vi "head.vi"(8 "error in (no error)":errorcluster, 11 "KNR in":T1) -> (0 "error out":errorcluster, 3 "KNR out":T1)   [LabVIEW 2013]
uses:
  <userlib>/KNR OS 3.0 LabVIEW Toolkit/Type Definition/KNR3 Reference.ctl
  <userlib>/_FPGA Interface Advanced Tools/FPGA Interface Base/FPGA Interface Base.lvclass
  <userlib>/KNR OS 3.0 LabVIEW Toolkit/Type Definition/Resource.ctl
  <userlib>/KNR OS 3.0 LabVIEW Toolkit/Type Definition/DC Motor Port.ctl
  Global 1.vi
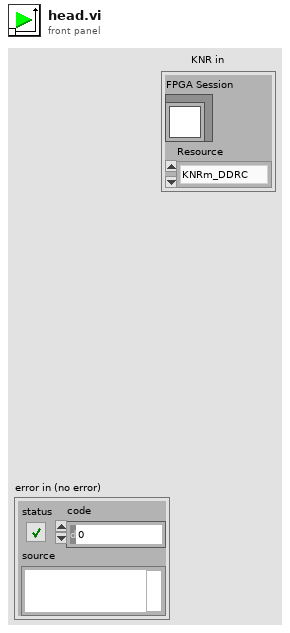
[diagram p1: front panel]
types:
  T1 = typedef "KNR3 Reference.ctl" = cluster{"FPGA Session":refnum<class "FPGA Interface Base.lvclass">, "Resource":T2}
  T2 = typedef "Resource.ctl" = enum16{"KNRm_DDRC", "KNRm_DDDD", "KNRm_DDDR", "KNRm_DDDC", "KNR"}
  T3 = typedef "DC Motor Port.ctl" = u16
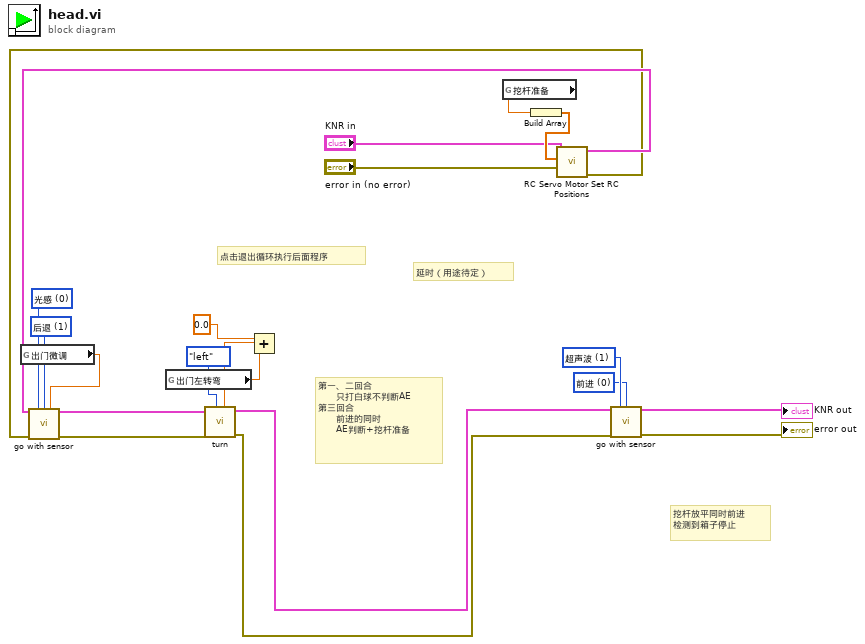
[diagram p0: block diagram]
diagram:
  w18 = T3 0 items=["前进", "后退"] ("方向")
  w19 = T3 1 items=["光感", "超声波"] ("传感器类型")
  w20 = T3 1 items=["前进", "后退"] ("方向")
  w12 = T3 0 items=["光感", "超声波"] ("传感器类型")
  # "第一、二回合\n      只打白球不判断AE\n第三回合\n      前进的同时\n      AE判断+挖杆准备"
  # "挖杆放平同时前进\n检测到箱子停止"
  # "延时（用途待定）"
  # "点击退出循环执行后面程序"
  n1 = global read "Global 1.vi" "出门微调"() -> (w11:dbl)
  n2 = global read "Global 1.vi" "出门左转弯"() -> (w14:dbl)
  n3 = Add(x=0.0, y=w14) -> (x+y=w13:dbl)
  n4 = global read "Global 1.vi" "挖杆准备"() -> (w6:dbl)
  n5 = Build Array(w6) -> (w5:dbl[])
  n6 = call <userlib>:"RC Servo Motor Set RC Positions.vi"("error in (no error)"="error in (no error)", "RC Pulse Width (1500 uS)"=w5, "KNR in"="KNR in") -> ("error out"=w3:errorcluster, "KNR out"=w4:T1)  [unwired: 7 in]
  n7 = call "go with sensor.vi"("KNR in"=w4, "传感器类型"=w12, "方向"=w20, "then go:"=w11, "error in (no error)"=w3) -> ("KNR out"=w10:T1, "error out"=w9:errorcluster)  [unwired: 8 in, 1 out]
  n8 = call "turn.vi"("Angle"=w13, "side"=enum16{"right", "left"}."left", "error in (no error)"=w9, "KNR in"=w10) -> ("error out"=w7:errorcluster, "KNR out"=w8:T1)  [unwired: 6 in]
  n9 = call "go with sensor.vi"("KNR in"=w8, "传感器类型"=w19, "方向"=w18, "error in (no error)"=w7) -> ("KNR out"=→"KNR out":T1, "error out"=→"error out":errorcluster)  [unwired: 9 in, 1 out]
